vi "Get ESP.vi"(8 "error in (no error)":errorcluster, 11 "ESP Actor in":refnum<class "ESP Actor.lvclass">) -> (0 "error out":errorcluster, 2 "ESP":bool, 3 "ESP Actor out":refnum<class "ESP Actor.lvclass">)   [LabVIEW 2020, in "ESP Actor.lvlib" / "ESP Actor.lvclass"]
uses:
  ESP Actor.lvclass
  ESP Actor.lvclass/ESP Actor.ctl
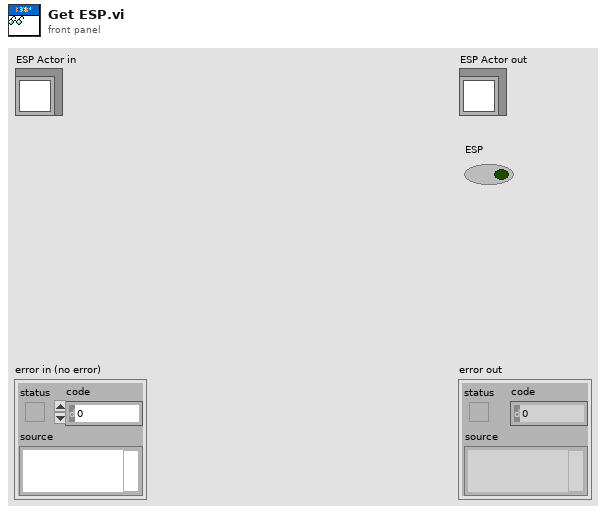
[diagram p1: front panel]
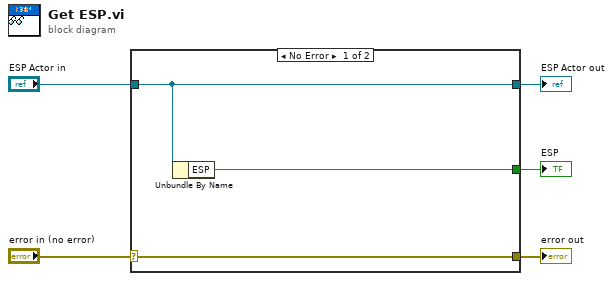
[diagram p0: block diagram]
diagram:
  n1 = case shown="No Error" "error in (no error)" {
    selector: "error in (no error)" -> [w8 w9]
    tunnel: [w8 w9] -> w4
    tunnel: [w7 w10] -> w2
    tunnel: "ESP Actor in" -> [w7 w10]
    tunnel: [w6 _] -> w1
    frame No Error {
      n2 = Unbundle By Name(w7) -> ("ESP"=w6:bool)
    }
    frame Error {
    }
  }
  "error out" <- w4
  "ESP Actor out" <- w2
  "ESP" <- w1
